vi "TDC_configureSyncDivider.vi"(8 "Error In":errorcluster, 10 "Reconstruct":bool, 11 "Divider":i32) -> (0 "Error Out":errorcluster)   [LabVIEW 2011]
uses:
  tdcbase.dll
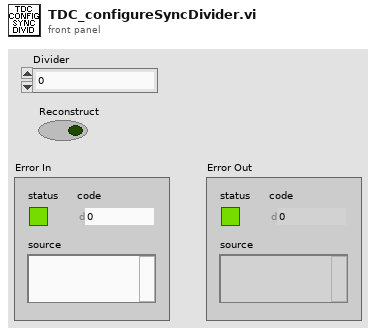
[diagram p1: front panel]
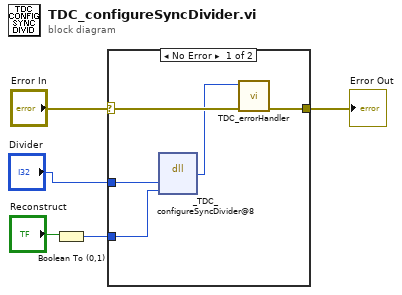
[diagram p0: block diagram]
diagram:
  n1 = Boolean To (0,1)(Boolean="Reconstruct") -> (0, 1=w1:i16)
  n2 = case shown="No Error" "Error In" {
    selector: "Error In" -> [w10 w11]
    tunnel: [w9 w11] -> w4
    tunnel: "Divider" -> [w7 _]
    tunnel: w1 -> [w6 _]
    frame No Error {
      n3 = dll-call lib="X:/tdcbase.dll" fn="_TDC_configureSyncDivider@8"("divider"=w7, "reconstruct"=w6) -> ("return type"=w8:i32)  [unwired: 5 in, 2 out]
      n4 = call "TDC_errorHandler.vi"("Error In"=w10, "TDC Return Code"=w8) -> ("Error Out"=w9:errorcluster)  [unwired: 9 in]
    }
    frame Error {
    }
  }
  "Error Out" <- w4
